vi "Send.vi"(10 "Helper Loop":refnum<class "Helper Loop.lvclass">) -> (3 "Helper Loop Create Msg out":refnum<class "Helper Loop Create Msg.lvclass">)   [LabVIEW 2021, in "Helper Loop Create.lvlib" / "Helper Loop Create Msg.lvclass"]
uses:
  Helper Loop Create Msg.lvclass
  Helper Loop/Helper Loop.lvclass
  Helper Loop Create Msg.lvclass/Helper Loop Create Msg.ctl
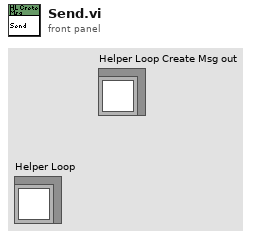
[diagram p1: front panel]
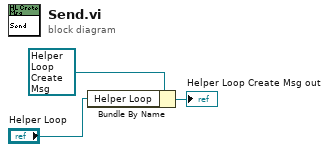
[diagram p0: block diagram]
diagram:
  n1 = Bundle By Name(cluster=refnum<class "Helper Loop Create Msg.lvclass"> refnum ("Panel Create Msg Strategy out"), "Helper Loop"="Helper Loop") -> (→"Helper Loop Create Msg out":refnum<class "Helper Loop Create Msg.lvclass">)
